vi "HFRR ADV v07.vi"() -> ()   [LabVIEW 2025] (continued)
                            n2274 = local write "EVENT LOG"(w3532) -> ()
                          }
                          frame Enabled {
                          }
                        }
                      }
                      frame #4 {
                        n2275 = Wait (ms)(milliseconds to wait=u32 50) -> ()  [unwired: 1 out]
                      }
                      frame #5 {
                        n2276 = local read "FILE"() -> (w3535:string)
                        n2277 = Concatenate Strings("File Name :" ("Content"), w3535) -> (w3536:string)
                        n2278 = local read "EVENT LOG"() -> (w3539:string)
                        n2279 = call "Event Log.vi"("Content"=w3536, "EVENT LOG"=w3539) -> ("EVENT LOG"=w3538:string)  [unwired: 8 in, 1 out]
                        n2280 = local write "EVENT LOG"(w3538) -> ()
                      }
                      frame #6 {
                        n2281 = Wait (ms)(milliseconds to wait=u32 50) -> ()  [unwired: 1 out]
                      }
                      frame #7 {
                        n2282 = local read "Batch Ref Num :"() -> (w3541:string)
                        n2283 = Concatenate Strings("Batch Ref No :" ("Content"), w3541) -> (w3542:string)
                        n2284 = local read "EVENT LOG"() -> (w3545:string)
                        n2285 = call "Event Log.vi"("Content"=w3542, "EVENT LOG"=w3545) -> ("EVENT LOG"=w3544:string)  [unwired: 8 in, 1 out]
                        n2286 = local write "EVENT LOG"(w3544) -> ()
                      }
                      frame #8 {
                        n2287 = Wait (ms)(milliseconds to wait=u32 50) -> ()  [unwired: 1 out]
                      }
                      frame #9 {
                        n2288 = local read "tested by"() -> (w3547:string)
                        n2289 = Concatenate Strings("Tested By :" ("Content"), w3547) -> (w3548:string)
                        n2290 = local read "EVENT LOG"() -> (w3551:string)
                        n2291 = call "Event Log.vi"("Content"=w3548, "EVENT LOG"=w3551) -> ("EVENT LOG"=w3550:string)  [unwired: 8 in, 1 out]
                        n2292 = local write "EVENT LOG"(w3550) -> ()
                      }
                      frame #10 {
                        n2293 = Wait (ms)(milliseconds to wait=u32 50) -> ()  [unwired: 1 out]
                      }
                      frame #11 {
                        n2294 = local read "TEST STANDARD"() -> (w3554:T4)
                        n2295 = case shown="\"ASTM D6079\", Default" w3554 {
                          tunnel: ["ASTM D6079" "ISO 12156" "CEC F-096-A-06" "Custom"] -> w3553
                          frame "ASTM D6079", Default {
                          }
                          frame "ISO 12156" {
                          }
                          frame "CEC F-096-A-06" {
                          }
                          frame "Custom" {
                          }
                        }
                        n2296 = Concatenate Strings("Test Standard :" ("Content"), w3553) -> (w3555:string)
                        n2297 = local read "EVENT LOG"() -> (w3558:string)
                        n2298 = call "Event Log.vi"("Content"=w3555, "EVENT LOG"=w3558) -> ("EVENT LOG"=w3557:string)  [unwired: 8 in, 1 out]
                        n2299 = local write "EVENT LOG"(w3557) -> ()
                      }
                      frame #12 {
                        n2300 = Wait (ms)(milliseconds to wait=u32 50) -> ()  [unwired: 1 out]
                      }
                      frame #13 {
                        n2301 = local read "Fuel Discription :"() -> (w3564:string)
                        n2302 = Concatenate Strings("Fuel Description :" ("Content"), w3564) -> (w3565:string)
                        n2303 = local read "EVENT LOG"() -> (w3568:string)
                        n2304 = call "Event Log.vi"("Content"=w3565, "EVENT LOG"=w3568) -> ("EVENT LOG"=w3567:string)  [unwired: 8 in, 1 out]
                        n2305 = local write "EVENT LOG"(w3567) -> ()
                      }
                      frame #14 {
                        n2306 = Wait (ms)(milliseconds to wait=u32 50) -> ()  [unwired: 1 out]
                      }
                      frame #15 {
                        n2307 = local read "Remarks :"() -> (w3570:string)
                        n2308 = Concatenate Strings("Remarks :" ("Content"), w3570) -> (w3571:string)
                        n2309 = local read "EVENT LOG"() -> (w3574:string)
                        n2310 = call "Event Log.vi"("Content"=w3571, "EVENT LOG"=w3574) -> ("EVENT LOG"=w3573:string)  [unwired: 8 in, 1 out]
                        n2311 = local write "EVENT LOG"(w3573) -> ()
                      }
                      frame #16 {
                        n2312 = Wait (ms)(milliseconds to wait=u32 50) -> ()  [unwired: 1 out]
                      }
                      frame #17 {
                        n2313 = local read "Operator ID"() -> (w3576:string)
                        n2314 = Concatenate Strings("Operator ID :" ("Content"), w3576) -> (w3578:string)
                        n2315 = local read "EVENT LOG"() -> (w3580:string)
                        n2316 = call "Event Log.vi"("Content"=w3578, "EVENT LOG"=w3580) -> ("EVENT LOG"=w3579:string)  [unwired: 8 in, 1 out]
                        n2317 = local write "EVENT LOG"(w3579) -> ()
                      }
                      frame #18 {
                        n2318 = Wait (ms)(milliseconds to wait=u32 50) -> ()  [unwired: 1 out]
                      }
                      frame #19 {
                        n2319 = disable-structure shown="Disabled" {
                          frame Disabled {
                            n2320 = local read "EVENT LOG"() -> (w3584:string)
                            n2321 = call "Event Log.vi"("Content"="Test Parameter", "EVENT LOG"=w3584) -> ("EVENT LOG"=w3583:string)  [unwired: 8 in, 1 out]
                            n2322 = local write "EVENT LOG"(w3583) -> ()
                          }
                          frame Enabled {
                          }
                        }
                      }
                      frame #20 {
                        n2323 = Wait (ms)(milliseconds to wait=u32 50) -> ()  [unwired: 1 out]
                      }
                      frame #21 {
                        n2324 = local read "Set Hz"() -> (w3588:dbl)
                        n2325 = Number To Fractional String(number=w3588, precision (6)=i16 2) -> (F-format string=w3587:string)  [unwired: 2 in]
                        n2326 = Concatenate Strings("Set Frequency [Hz] :" ("Content"), w3587) -> (w3590:string)
                        n2327 = local read "EVENT LOG"() -> (w3592:string)
                        n2328 = call "Event Log.vi"("Content"=w3590, "EVENT LOG"=w3592) -> ("EVENT LOG"=w3591:string)  [unwired: 8 in, 1 out]
                        n2329 = local write "EVENT LOG"(w3591) -> ()
                      }
                      frame #22 {
                        n2330 = Wait (ms)(milliseconds to wait=u32 50) -> ()  [unwired: 1 out]
                      }
                      frame #23 {
                        n2331 = local read "NORMAL LOAD"() -> (w3595:dbl)
                        n2332 = Number To Fractional String(number=w3595, precision (6)=i16 2) -> (F-format string=w3596:string)  [unwired: 2 in]
                        n2333 = Concatenate Strings("Applied Load [N] :" ("Content"), w3596) -> (w3598:string)
                        n2334 = local read "EVENT LOG"() -> (w3600:string)
                        n2335 = call "Event Log.vi"("Content"=w3598, "EVENT LOG"=w3600) -> ("EVENT LOG"=w3599:string)  [unwired: 8 in, 1 out]
                        n2336 = local write "EVENT LOG"(w3599) -> ()
                      }
                      frame #24 {
                        n2337 = Wait (ms)(milliseconds to wait=u32 50) -> ()  [unwired: 1 out]
                      }
                      frame #25 {
                        n2338 = local read "Set Strk"() -> (w3603:dbl)
                        n2339 = Number To Fractional String(number=w3603, precision (6)=i16 2) -> (F-format string=w3604:string)  [unwired: 2 in]
                        n2340 = Concatenate Strings("Set Stroke [mm] :" ("Content"), w3604) -> (w3606:string)
                        n2341 = local read "EVENT LOG"() -> (w3608:string)
                        n2342 = call "Event Log.vi"("Content"=w3606, "EVENT LOG"=w3608) -> ("EVENT LOG"=w3607:string)  [unwired: 8 in, 1 out]
                        n2343 = local write "EVENT LOG"(w3607) -> ()
                      }
                      frame #26 {
                        n2344 = Wait (ms)(milliseconds to wait=u32 50) -> ()  [unwired: 1 out]
                      }
                      frame #27 {
                        n2345 = local read "Set Temp"() -> (w3611:dbl)
                        n2346 = Number To Fractional String(number=w3611, precision (6)=i16 2) -> (F-format string=w3612:string)  [unwired: 2 in]
                        n2347 = Concatenate Strings("Set Temperature [deg C] :" ("Content"), w3612) -> (w3614:string)
                        n2348 = local read "EVENT LOG"() -> (w3616:string)
                        n2349 = call "Event Log.vi"("Content"=w3614, "EVENT LOG"=w3616) -> ("EVENT LOG"=w3615:string)  [unwired: 8 in, 1 out]
                        n2350 = local write "EVENT LOG"(w3615) -> ()
                      }
                      frame #28 {
                        n2351 = Wait (ms)(milliseconds to wait=u32 50) -> ()  [unwired: 1 out]
                      }
                      frame #29 {
                        n2352 = local read "Set Rh"() -> (w3619:dbl)
                        n2353 = Number To Fractional String(number=w3619, precision (6)=i16 2) -> (F-format string=w3620:string)  [unwired: 2 in]
                        n2354 = Concatenate Strings("Set Humidity [%RH] :" ("Content"), w3620) -> (w3622:string)
                        n2355 = local read "EVENT LOG"() -> (w3624:string)
                        n2356 = call "Event Log.vi"("Content"=w3622, "EVENT LOG"=w3624) -> ("EVENT LOG"=w3623:string)  [unwired: 8 in, 1 out]
                        n2357 = local write "EVENT LOG"(w3623) -> ()
                      }
                      frame #30 {
                        n2358 = Wait (ms)(milliseconds to wait=u32 50) -> ()  [unwired: 1 out]
                      }
                      frame #31 {
                        n2359 = local read "test time"() -> (w3627:dbl)
                        n2360 = Number To Fractional String(number=w3627, precision (6)=i16 1) -> (F-format string=w3628:string)  [unwired: 2 in]
                        n2361 = Concatenate Strings("Test Time [mins] :" ("Content"), w3628) -> (w3630:string)
                        n2362 = local read "EVENT LOG"() -> (w3632:string)
                        n2363 = call "Event Log.vi"("Content"=w3630, "EVENT LOG"=w3632) -> ("EVENT LOG"=w3631:string)  [unwired: 8 in, 1 out]
                        n2364 = local write "EVENT LOG"(w3631) -> ()
                      }
                    }
                  }
                }
              }
            }
          }
        }
        n2365 = case shown="True" w2932 {
          frame False {
            n2366 = local write "tfalg"(0.0 ("tfalg")) -> ()
          }
          frame True {
            n2367 = local read "tfalg"() -> (w3077:dbl)
            n2368 = Equal?(x=w3077, y=0.0) -> (x = y?=w3078:bool)
            n2369 = case shown="True" w3078 {
              frame False {
              }
              frame True {
                n2370 = local read "Total No. of Tests"() -> (w3081:dbl)
                n2371 = local write "tfalg"(1.0 ("tfalg")) -> ()
                n2372 = local write "acq 2"(FALSE ("acq 2")) -> ()
                n2373 = Wait (ms)(milliseconds to wait=u32 200) -> ()  [unwired: 1 out]
                n2374 = Increment(x=w3081) -> (x+1=w3080:dbl)
                n2375 = local write "Total No. of Tests"(w3080) -> ()
              }
            }
          }
        }
        n2376 = local write "Test \nStatus"(w2938) -> ()
        n2377 = local write "st enable"(w2938) -> ()
        n2378 = local write "PWR"(w2938) -> ()
        n2379 = local write "Save"(w2938) -> ()
        n2380 = local read "Main Tab"() -> (w2895:T3)
        n2381 = case shown="True" w2919 {
          tunnel: [FALSE ("RUN") TRUE ("RUN")] -> w2918
          tunnel: [_ 1] -> w2911
          frame False {
          }
          frame True {
          }
        }
        n2382 = In Range and Coerce(upper limit=w2926, x=w2899, lower limit=w2925) -> (In Range?=w2917:bool)  [unwired: 1 out]
        n2383 = In Range and Coerce(upper limit=w2923, x=w2898, lower limit=w2924) -> (In Range?=w2915:bool)  [unwired: 1 out]
        n2384 = case shown="True" w2931 {
          frame False {
            n2385 = local read "Rt 3"() -> (w3059:bool)
            n2386 = case shown="True" w3059 {
              frame False {
              }
              frame True {
                n2387 = local write "Rt 3"(FALSE ("Rt 3")) -> ()
                n2388 = local write "Json End Flg"(TRUE ("Upld AR 2")) -> ()
              }
            }
            "Rt" <- TRUE ("Rt")
            "Rt 2" <- FALSE ("Rt")
          }
          frame True {
            n2389 = local read "Rt"() -> (w3066:bool)
            n2390 = local write "Rt 2"(TRUE ("Rt 2")) -> ()
            n2391 = case shown="True" w3066 {
              frame False {
              }
              frame True {
                w3067 = TRUE ("Upld AR 2")
                n2392 = local write "Rt"(FALSE ("Rt")) -> ()
                n2393 = local write "Upld AR"(w3067) -> ()
                n2394 = local write "Json St Flg"(w3067) -> ()
              }
            }
            "Rt 3" <- TRUE ("Rt 3")
          }
        }
        n2395 = case shown="True" w2917 {
          tunnel: [FALSE ("RUN") TRUE ("RUN")] -> w2916
          tunnel: [_ 2] -> w2910
          frame False {
          }
          frame True {
          }
        }
        n2396 = case shown="True" w2915 {
          tunnel: [FALSE ("RUN") TRUE ("RUN")] -> w2914
          tunnel: [_ 3] -> w2909
          frame False {
          }
          frame True {
          }
        }
        n2397 = case shown="\"Acquire\"" w2895 {
          tunnel: w2897 -> [_ w3128]
          frame Default {
            w3127 = 0.0 ("output")
            n2398 = local write "PID-out"(w3127) -> ()
            n2399 = local write "Frequency ( Hz )"(w3127) -> ()
          }
          frame "Acquire" {
            n2400 = stacked-sequence {
              frame #0 {
                n2401 = local read "Auto Start Test"() -> (w3130:bool)
                n2402 = case shown="False" w3130 {
                  tunnel: "RUN" -> [w3151 w3154]
                  tunnel: [w3151 w3153] -> w3131
                  frame False {
                  }
                  frame True {
                    n2403 = local read "Auto Start Temp"() -> (w3152:bool)
                    n2404 = Or(x=w3154, y=w3152) -> (x .or. y?=w3153:bool)
                  }
                }
                n2405 = local read "clk"() -> (w3150:dbl)
                n2406 = local read "Save"() -> (w3146:bool)
                n2407 = Equal?(x=w3150, y=0.0) -> (x = y?=w3147:bool)
                n2408 = And(x=w3147, y=w3146) -> (x .and. y?=w3148:bool)
                n2409 = Not(x="Engage") -> (.not. x?=w3137:bool)
                n2410 = case shown="False" w3131 {
                  tunnel: [w3163 w3179] -> w3133
                  frame False {
                    w3163 = 0.0
                    n2411 = local write "Reinit PID"(TRUE) -> ()
                    n2412 = local write "Start Time"(TRUE ("Start Time")) -> ()
                    n2413 = property on="Stroke" class="DigNum (strict)"("Visible"=TRUE) -> ()  [unwired: 2 in, 2 out]
                    n2414 = property on="Stroke 2" class="DigNum (strict)"("Visible"=FALSE) -> ()  [unwired: 2 in, 2 out]
                    n2415 = property on="Heater Button" class="Bool (strict)"("DisabledEnum"=T15."Enabled" ("Disabled")) -> ()  [unwired: 2 in, 2 out]
                    n2416 = property on="Humidity" class="Bool (strict)"("DisabledEnum"=T15."Enabled" ("Disabled")) -> ()  [unwired: 2 in, 2 out]
                    n2417 = case shown="False" "TestCompFlg" {
                      frame False {
                        n2418 = local read "StartFlg"() -> (w3167:bool)
                        n2419 = case shown="True" w3167 {
                          frame False {
                          }
                          frame True {
                            n2420 = flat-sequence {
                              frame #0 {
                                n2421 = local read "EVENT LOG"() -> (w3169:string)
                                n2422 = call "Event Log.vi"("Content"="Test was interrupted", "EVENT LOG"=w3169) -> ("EVENT LOG"=w3170:string)  [unwired: 8 in, 1 out]
                                n2423 = local write "EVENT LOG"(w3170) -> ()
                              }
                              frame #1 {
                                w3171 = FALSE ("StartFlg")
                                n2424 = local write "Heater Button"(w3171) -> ()
                                n2425 = local write "StartFlg"(w3171) -> ()
                                n2426 = local write "Humidity"(w3171) -> ()
                              }
                            }
                          }
                        }
                      }
                      frame True {
                      }
                    }
                    n2427 = local write "String 14"("Test will autostart once parameters reach the set value." ("String 14")) -> ()
                    n2428 = local write "Old Pid Val"(w3163) -> ()
                  }
                  frame True {
                    n2429 = property on="Stroke 2" class="DigNum (strict)"("Visible"=TRUE) -> ()  [unwired: 2 in, 2 out]
                    n2430 = property on="Stroke" class="DigNum (strict)"("Visible"=FALSE) -> ()  [unwired: 2 in, 2 out]
                    n2431 = property on="STOP 2" class="Bool (strict)"("Disabled"=u8 2) -> ()  [unwired: 2 in, 2 out]
                    n2432 = local write "String 14"(" Running....." ("String 14")) -> ()
                    n2433 = property on="Heater Button" class="Bool (strict)"("DisabledEnum"=T15."Disabled and Grayed Out" ("Disabled")) -> ()  [unwired: 2 in, 2 out]
                    n2434 = property on="Humidity" class="Bool (strict)"("DisabledEnum"=T15."Disabled and Grayed Out" ("Disabled")) -> ()  [unwired: 2 in, 2 out]
                    n2435 = local read "PID Ref"() -> (w3190:bool)
                    n2436 = case shown="True" w3190 {
                      tunnel: [w3196 w3212] -> w3189
                      frame False {
                        n2437 = local read "Old Pid Val"() -> (w3196:dbl)
                      }
                      frame True {
                        n2438 = local read "Set Hz"() -> (w3205:dbl)
                        n2439 = local read "Frequency"() -> (w3216:dbl)
                        n2440 = Add(x=w3205, y=10.0) -> (x+y=w3214:dbl)
                        n2441 = Add(x=w3205, y=-10.0 ("Offset")) -> (x+y=w3223:dbl)
                        n2442 = Add(x=w3205, y=-10.0) -> (x+y=w3215:dbl)
                        n2443 = In Range and Coerce(upper limit=w3214, x=w3216, lower limit=w3215) -> (coerced(x)=w3204:dbl)  [unwired: 1 out]
                        n2444 = Or(x="Reinit PID", y="Reinit PID") -> (x .or. y?=w3213:bool)
                        n2445 = Multiply(x=w3223, y=0.1 ("Gain")) -> (x*y=w3202:dbl)
                        n2446 = local read "Elapsed time"() -> (w3209:dbl)
                        n2447 = local read "SPEED OUT:"() -> (w3224:dbl)
                        n2448 = Add(x=w3202, y=1.5) -> (x+y=w3200:dbl)
                        n2449 = call-poly <vilib>:"PID.vi"("reinitialize? (F)"=w3213, "output range"=cluster{"output high":dbl, "output low":dbl} {"output high"=1.0, "output low"=-1.0}, "PID gains"=T11 {"proportional gain (Kc)"=0.0005, "integral time (Ti, min)"=0.001, "derivative time (Td, min)"=0.0} ("Motor PID"), "process variable"=w3204, "setpoint"=w3205) -> ("output"=w3203:dbl)  [unwired: 5 in, 1 out]
                        n2450 = Multiply(x=w3200, y=w3224) -> (x*y=w3199:dbl)
                        n2451 = Greater?(x=w3209, y=0.05) -> (0:w3208:bool)
                        n2452 = case shown="True" w3208 {
                          tunnel: w3203 -> [_ w3226]
                          tunnel: [0.0 ("output") w3226] -> w3206
                          frame False {
                          }
                          frame True {
                            n2453 = local write "Reinit PID"(FALSE ("Reinit PID")) -> ()
                          }
                        }
                        n2454 = Multiply(x=w3199, y=0.8) -> (x*y=w3198:dbl)
                        n2455 = Add(x=w3198, y=w3206) -> (x+y=w3211:dbl)
                        n2456 = flat-sequence {
                          tunnel: [w3229] -> w3212
                          tunnel: w3211 -> [w3229]
                          frame #0 {
                            n2457 = local write "PID Ref"(FALSE ("PID Ref")) -> ()
                          }
                        }
                      }
                    }
                    "Old Pid Val" <- w3189
                    n2458 = case shown="False" "Start Time" {
                      selector: "Start Time" -> [_ w3192]
                      frame False {
                      }
                      frame True {
                        n2459 = Not(x=w3192) -> (.not. x?=w3191:bool)
                        n2460 = local write "Start Time"(w3191) -> ()
                        n2461 = local read "EVENT LOG"() -> (w3193:string)
                        n2462 = call "Event Log.vi"("Content"="Test in progress", "EVENT LOG"=w3193) -> ("EVENT LOG"=w3195:string)  [unwired: 8 in, 1 out]
                        n2463 = local write "EVENT LOG"(w3195) -> ()
                      }
                    }
                    n2464 = local read "Set Hz"() -> (w3186:dbl)
                    n2465 = call <vilib>:"Uniform White Noise Waveform.vi"() -> ("signal out"=w3185:waveform(dbl))  [unwired: 10 in, 1 out]
                    n2466 = local read "Freq"() -> (w3178:dbl)
                    n2467 = Add(x=w3186, y=w3185) -> (x+y=w3184:waveform(dbl))
                    n2468 = Multiply(x=w3184, y=ext 0.1) -> (x*y=w3180:waveform(ext))
                    n2469 = Multiply(x=w3178, y=0.9) -> (x*y=w3181:dbl)
                    n2470 = Add(x=w3180, y=w3181) -> (x+y=w3179:waveform(ext))
                    "StartFlg" <- TRUE ("StartFlg")
                  }
                }
                n2471 = case shown="True" w3148 {
                  frame False {
                  }
                  frame True {
                    n2472 = local write "clk"(10.0 ("clk")) -> ()
                    n2473 = Get Date/Time In Seconds() -> (seconds since 1Jan1904=w3232:timestamp)
                    n2474 = To Double Precision Float(number=w3232) -> (double precision float=w3230:dbl)
                    n2475 = local write "acq timer"(w3230) -> ()
                    n2476 = local write "act save time"(w3230) -> ()
                  }
                }
                n2477 = call "Elapsed Time"("Time Target (s)"="Countdown", "Reset"=w3137) -> ("Elapsed Time (s)"=w3142:dbl, "Time has Elapsed"=w3140:bool)  [unwired: 10 in, 6 out]
                "Countdown 2" <- w3142
                n2478 = Subtract(x=w3142, y=2.0) -> (x-y=w3145:dbl)
                n2479 = Less?(x=w3145, y="Countdown") -> (x < y?=w3143:bool)
                n2480 = And(x=w3143, y=w3140) -> (x .and. y?=w3139:bool)
                n2481 = case shown="True" w3139 {
                  frame False {
                  }
                  frame True {
                    (unwired) dbl[] [] ("History Data")
                    n2482 = local write "Engage"(FALSE ("Engage")) -> ()
                    n2483 = local write "RUN"(TRUE ("RUN")) -> ()
                    n2484 = local read "Humidity ( %RH )"() -> (→"Rh Before":dbl)
                  }
                }
                n2485 = local read "Test \nStatus"() -> (w3135:bool)
                n2486 = Select(t=w3133, s=w3135, f=0.0) -> (s? t:f=w3134:dbl)
                n2487 = local write "Frequency ( Hz )"(w3134) -> ()
                n2488 = local write "Freq"(w3134) -> ()
              }
              frame #1 {
                w3255 = 1000000.0 ("x")
                # "Elapsed time\ncof\nstroke\nAir temp\nTemp\nHumidity"
                # "acq timer\n\nact save time"
                # "convert to microseconds"
                n2489 = local read "COUNT"() -> (w3238:i32)
                n2490 = local read "Rate"() -> (w3251:dbl)
                n2491 = Divide(x=w3255, y=w3251) -> (x/y=w3256:dbl)
                n2492 = Greater Or Equal?(x=w3238, y=250) -> (x >= y?=w3237:bool)
                n2493 = Get Date/Time In Seconds() -> (seconds since 1Jan1904=w3258:timestamp)
                n2494 = case shown="True" w3237 {
                  frame False {
                    n2495 = local read "COUNT"() -> (w3259:i32)
                    n2496 = Increment(x=w3259) -> (x+1=w3260:i32)
                    n2497 = local write "COUNT"(w3260) -> ()
                  }
                  frame True {
                    n2498 = local write "COUNT"(0 ("COUNT")) -> ()
                  }
                }
                n2499 = local read "Samplingtime 2"() -> (w3236:dbl)
                n2500 = local read "act save time"() -> (w3253:dbl)
                n2501 = Divide(x=w3256, y=w3255) -> (x/y=w3254:dbl)
                n2502 = To Double Precision Float(number=w3258) -> (double precision float=w3247:dbl)
                n2503 = Add(x=w3253, y=w3236) -> (x+y=w3252:dbl)
                n2504 = local read "acq timer"() -> (w3257:dbl)
                n2505 = local read "COUNT"() -> (w3240:i32)
                n2506 = Greater Or Equal?(x=w3247, y=w3252) -> (x >= y?=w3235:bool)
                n2507 = Multiply(x=w3254, y=w3240) -> (x*y=w3246:dbl)
                n2508 = Subtract(x=w3247, y=w3257) -> (x-y=w3249:dbl)
                n2509 = local read "Save"() -> (w3250:bool)
                n2510 = Add(x=w3249, y=w3246) -> (x+y=w3233:dbl)
                "Elapsed time 3" <- w3233
                n2511 = And(x=w3235, y=w3250) -> (x .and. y?=w3248:bool)
                n2512 = Divide(x=w3233, y=60.0) -> (x/y=w3244:dbl)
                n2513 = local read "Test \nStatus"() -> (w3234:bool)
                n2514 = local read "clk"() -> (w3241:dbl)
                n2515 = Equal?(x=w3241, y=10.0) -> (x = y?=w3243:bool)
                n2516 = case shown="True" w3248 {
                  tunnel: w3247 -> [_ w3354]
                  tunnel: [FALSE ("Boolean 2") TRUE ("Boolean 2")] -> _
                  frame False {
                  }
                  frame True {
                    w3301 = ";" ("Substring")
                    # "Pid out/\nFreq response value"
                    n2517 = local write "act save time"(w3354) -> ()
                    n2518 = local read "FILE"() -> (w3295:string)
                    n2519 = call "file check.vi"("file name in"=w3295) -> ("error out"=w3298:errorcluster, "file name out"=w3293:string)  [unwired: 9 in]
                    n2520 = call "FILE PATH CREATION.vi"("error in"=w3298, "FILE NAME :"=w3293) -> ("FILE OUT"=w3296:path)  [unwired: 8 in, 1 out]
                    n2521 = Concatenate Strings(w3293, ".dgf" ("Substring")) -> (w3297:string)
                    n2522 = local read "Set Strk"() -> (w3325:dbl)
                    n2523 = local read "Stroke"() -> (w3316:dbl)
                    n2524 = local read "FF 2"() -> (w3312:dbl)
                    "Frictional Force ( N )" <- w3312
                    "Frictional Force ( N )" <- w3312
                    n2525 = Build Path(base path=w3296, name or relative path=w3297) -> (appended path=w3292:path)
                    n2526 = local write "FF 3"(w3312) -> ()
                    n2527 = Subtract(x=w3316, y=w3325) -> (x-y=w3322:dbl)
                    n2528 = local read "COF 2"() -> (w3307:dbl)
                    "cof" <- w3307
                    "Coefficient of Friction" <- w3307
                    "COF 4" <- w3307
                    "Coefficient of Friction" <- w3307
                    n2529 = local write "COF 3"(w3307) -> ()
                    n2530 = Multiply(x=w3322, y=0.05) -> (x*y=w3324:dbl)
                    n2531 = local read "TEMP"() -> (w3311:dbl)
                    "Temp" <- w3311
                    "Temperature ( Deg C )" <- w3311
                    n2532 = Add(x=w3324, y=w3325) -> (x+y=w3305:dbl)
                    "Stroke Ln" <- w3305
                    "Disp" <- w3305
                    n2533 = local read "ecr"() -> (w3308:dbl)
                    "ecr 2" <- w3308
                    "Electrical Contact Resistance ( % )" <- w3308
                    "ecr 4" <- w3308
                    n2534 = local read "Humidity ( %RH )"() -> (w3310:dbl)
                    "Humidity ( %RH )" <- w3310
                    "Humidity ( %RH )" <- w3310
                    n2535 = local read "Frequency ( Hz )"() -> (w3318:dbl)
                    n2536 = local read "Elapsed time"() -> (w3347:dbl)
                    n2537 = local read "AIR TEMP"() -> (w3315:dbl)
                    n2538 = local write "ecr 3"(w3308) -> ()
                    n2539 = local read "PID-out"() -> (w3321:dbl)
                    n2540 = local write "Temperature ( Deg C )"(w3311) -> ()
                    n2541 = local write "Electrical Contact Resistance ( % )"(w3308) -> ()
                    n2542 = Number To Fractional String(number=w3305, width (-)=i16 9 ("precision (6)"), precision (6)=i16 6) -> (F-format string=w3340:string)  [unwired: 1 in]
                    n2543 = Number To Fractional String(number=w3315, width (-)=i16 9 ("precision (6)"), precision (6)=i16 3) -> (F-format string=w3339:string)  [unwired: 1 in]
                    n2544 = Number To Fractional String(number=w3311, width (-)=i16 9 ("precision (6)"), precision (6)=i16 3) -> (F-format string=w3336:string)  [unwired: 1 in]
                    n2545 = Number To Fractional String(number=w3310, width (-)=i16 9 ("precision (6)"), precision (6)=i16 3) -> (F-format string=w3333:string)  [unwired: 1 in]
                    n2546 = Number To Fractional String(number=w3308, width (-)=i16 9 ("precision (6)"), precision (6)=i16 3) -> (F-format string=w3330:string)  [unwired: 1 in]
                    n2547 = Number To Fractional String(number=w3321, width (-)=i16 9 ("precision (6)"), precision (6)=i16 3) -> (F-format string=w3326:string)  [unwired: 1 in]
                    n2548 = Number To Fractional String(number=w3318, width (-)=i16 9 ("precision (6)"), precision (6)=i16 3) -> (F-format string=w3317:string)  [unwired: 1 in]
                    n2549 = Number To Fractional String(number=w3307, width (-)=i16 9 ("precision (6)"), precision (6)=i16 6) -> (F-format string=w3348:string)  [unwired: 1 in]
                    n2550 = Number To Fractional String(number=w3347, width (-)=i16 14 ("precision (6)"), precision (6)=i16 3) -> (F-format string=w3349:string)  [unwired: 1 in]
                    n2551 = Bundle("y"=1.02, w3305, "y"=0.98) -> (w3309:cluster{"y":dbl, dbl, "y":dbl})  [unwired: 1 in]
                    n2552 = Number To Fractional String(number="Ambient Humidity :", width (-)=i16 9 ("precision (6)"), precision (6)=i16 6) -> (F-format string=w3299:string)  [unwired: 1 in]
                    n2553 = local read "RUN"() -> (w3306:bool)
                    n2554 = case shown="True" w3306 {
                      tunnel: w3309 -> [_ w3359]
                      tunnel: w3305 -> [_ w3358]
                      tunnel: w3305 -> [_ w3357]
                      tunnel: w3305 -> [_ w3356]
                      frame False {
                      }
                      frame True {
                        "Stroke ( mm )" <- w3359
                        "Stroke ( mm )" <- w3359
                        "Stroke 4" <- w3358
                        "Stroke 3" <- w3357
                        "Stroke 2" <- w3356
                      }
                    }
                    n2555 = Concatenate Strings(w3349, w3301, w3348, w3301, w3340, w3301, w3339, w3301, w3336, w3301, w3333, w3301, w3330, w3301, w3326, w3301, w3317, w3301, w3299, "\r") -> (w3346:string)
                    n2556 = call <vilib>:"Write Characters To File.vi"("append to file? (new file:F)"=TRUE, "character string"=w3346, "file path (dialog if empty)"=w3292) -> ()  [unwired: 2 in, 1 out]
                    "refresh flag" <- TRUE ("refresh flag")
                  }
                }
                n2557 = case shown="True" w3234 {
                  tunnel: w3244 -> [_ w3267]
                  tunnel: w3249 -> [_ w3278]
                  tunnel: [0.0 w3274] -> _
                  tunnel: w3243 -> [_ w3273]
                  tunnel: [0.0 w3272] -> _
                  tunnel: w3233 -> [_ w3272]
                  tunnel: w3247 -> [w3263 _]
                  frame False {
                    n2558 = local write "acq timer"(w3263) -> ()
                    n2559 = local write "Test Duration Status"(0.0 ("Test Duration Status")) -> ()
                  }
                  frame True {
                    n2560 = local read "Set Hz"() -> (w3275:dbl)
                    n2561 = local write "Elapsed time"(w3267) -> ()
                    n2562 = local read "test time"() -> (w3266:dbl)
                    n2563 = Multiply(x=w3278, y=w3275) -> (x*y=w3277:dbl)
                    n2564 = case shown="False" w3273 {
                      tunnel: w3277 -> [w3279 _]
                      tunnel: [w3279 1.0] -> w3274
                      frame False {
                        n2565 = local write "Cycles elapsed"(w3279) -> ()
                      }
                      frame True {
                      }
                    }
                    n2566 = Greater?(x=w3267, y=w3266) -> (0:w3276:bool)
                    n2567 = Subtract(x=w3266, y=w3267) -> (x-y=w3271:dbl)
                    "time" <- w3271
                    n2568 = local write "Time Remaining"(w3271) -> ()
                    n2569 = case shown="True" w3276 {
                      frame False {
                      }
                      frame True {
                        n2570 = local write "Humidity"(FALSE ("Humidity")) -> ()
                        n2571 = local write "RUN"(FALSE ("OK Button 2")) -> ()
                        n2572 = local write "Heater Button"(FALSE ("Heater Button")) -> ()
                        n2573 = local write "Auto Start Test"(FALSE ("Auto Start Test")) -> ()
                        n2574 = local write "TestCompFlg"(TRUE ("StpFlg")) -> ()
                        n2575 = local read "Humidity ( %RH )"() -> (→"Rh After":dbl)
                        n2576 = property on="STOP 2" class="Bool (strict)"("Disabled"=u8 0) -> ()  [unwired: 2 in, 2 out]
                        n2577 = local read "EVENT LOG"() -> (w3285:string)
                        n2578 = call "Event Log.vi"("Content"="Test Completed", "EVENT LOG"=w3285) -> ("EVENT LOG"=w3284:string)  [unwired: 8 in, 1 out]
                        n2579 = local write "EVENT LOG"(w3284) -> ()
                      }
                    }
                    n2580 = Divide(x=w3267, y=w3266) -> (x/y=w3270:dbl)
                    n2581 = Multiply(x=w3270, y=100.0) -> (x*y=w3268:dbl)
                    n2582 = local write "Test Duration Status"(w3268) -> ()
                  }
                }
              }
              frame #2 {
                n2583 = case shown="True" "Heater Button" {
                  tunnel: [0.0 ("output") w3383] -> w3360
                  frame False {
                    w3363 = TRUE ("tmpchk")
                    n2584 = local read "TEMP"() -> (w3364:dbl)
                    n2585 = local write "Temp ini"(w3364) -> ()
                    n2586 = local write "Reset 4"(w3363) -> ()
                    n2587 = local write "tmpchk"(w3363) -> ()
                    n2588 = local write "reinit"(TRUE ("reinit")) -> ()
                    n2589 = local write "manual temp log"(TRUE ("manual temp log")) -> ()
                  }
                  frame True {
                    # "Logic to turn off\nthe heater when \ntemp is not rising.\nTime - 60 sec\nDelta t- 5°c"
                    n2590 = local read "Temp ini"() -> (w3371:dbl)
                    n2591 = local read "Auto Start Test"() -> (w3367:bool)
                    n2592 = Less?(x=w3371, y=53.0) -> (x < y?=w3369:bool)
                    n2593 = case shown="False" w3367 {
                      frame False {
                        n2594 = local read "Set Temp"() -> (w3394:dbl)
                        n2595 = local read "TEMP"() -> (w3393:dbl)
                        n2596 = Subtract(x=w3394, y=w3393) -> (x-y=w3392:dbl)
                        n2597 = Absolute Value(x=w3392) -> (abs(x)=w3391:dbl)
                        n2598 = Less?(x=w3391, y=0.5) -> (x < y?=w3389:bool)
                        n2599 = case shown="True" w3389 {
                          tunnel: "manual temp log" -> [_ w3395]
                          frame False {
                          }
                          frame True {
                            n2600 = case shown="True" w3395 {
                              selector: w3395 -> [_ w3396]
                              frame False {
                              }
                              frame True {
                                # "#Event log"
                                n2601 = Not(x=w3396) -> (.not. x?=w3397:bool)
                                n2602 = local write "manual temp log"(w3397) -> ()
                                n2603 = local read "EVENT LOG"() -> (w3400:string)
                                n2604 = call "Event Log.vi"("Content"="Target Temperature reached", "EVENT LOG"=w3400) -> ("EVENT LOG"=w3399:string)  [unwired: 8 in, 1 out]
                                n2605 = local write "EVENT LOG"(w3399) -> ()
                              }
                            }
                          }
                        }
                      }
                      frame True {
                        n2606 = local write "manual temp log"(TRUE ("manual temp log")) -> ()
                      }
                    }
                    n2607 = And(x="tmpchk", y=w3369) -> (x .and. y?=w3372:bool)
                    n2608 = case shown="True" w3372 {
                      frame False {
                      }
                      frame True {
                        n2609 = call "Elapsed Time8"("Time Target (s)"=300.0, "Reset"="Reset 4") -> ("Time has Elapsed"=w3402:bool)  [unwired: 10 in, 7 out]
                        n2610 = flat-sequence {
                          tunnel: w3402 -> [_]
                          frame #0 {
                            n2611 = local write "Reset 4"(FALSE ("Reset 4")) -> ()
                          }
                        }
                        n2612 = case shown="True" w3402 {
                          frame False {
                          }
                          frame True {
                            n2613 = local read "Temp ini"() -> (w3409:dbl)
                            n2614 = Add(x=w3409, y=5.0) -> (x+y=w3407:dbl)
                            n2615 = local read "TEMP"() -> (w3410:dbl)
                            n2616 = Greater?(x=w3410, y=w3407) -> (0:w3408:bool)
                            n2617 = case shown="False" w3408 {
                              frame False {
                                n2618 = local write "Heater Button"(FALSE ("Heater Button")) -> ()
                              }
                              frame True {
                                n2619 = local write "tmpchk"(FALSE ("tmpchk")) -> ()
                              }
                            }
                          }
                        }
                      }
                    }
                    n2620 = local read "Set Temp"() -> (w3380:dbl)
                    n2621 = local read "TEMP"() -> (w3374:dbl)
                    n2622 = call-poly <vilib>:"PID.vi"("reinitialize? (F)"="reinit", "output range"="output range", "dt (s)"=-1.0, "PID gains"="Temp PID gains", "process variable"=w3374, "setpoint"=w3380) -> ("output"=w3377:dbl)  [unwired: 4 in, 1 out]
                    n2623 = Subtract(x=w3380, y=w3374) -> (x-y=w3382:dbl)
                    n2624 = Add(x=w3380, y=0.5) -> (x+y=w3378:dbl)
                    n2625 = Greater Or Equal?(x=w3374, y=w3378) -> ()  [unwired: 1 out]
                    n2626 = Select(t=0.0, s=FALSE, f=w3377) -> (s? t:f=w3376:dbl)
                    "PID output" <- w3376
                    n2627 = flat-sequence {
                      tunnel: w3376 -> [w3413]
                      tunnel: [w3413] -> w3383
                      frame #0 {
                        n2628 = local write "reinit"(FALSE ("reinit")) -> ()
                      }
                    }
                    n2629 = Bundle(w3382, "output"=w3376, "TEMP"=w3374) -> (→"gTEMP 3":cluster{dbl, "output":dbl, "TEMP":dbl})  [unwired: 1 in]
                  }
                }
                "PID-out" <- w3360
              }
              frame #3 {
                n2630 = local read "TEMP"() -> (w3415:dbl)
                n2631 = Greater Or Equal?(x=w3415, y="Set Temp 2") -> (x >= y?=w3420:bool)
                n2632 = case shown="True" w3420 {
                  tunnel: [FALSE TRUE] -> w3418
                  frame False {
                  }
                  frame True {
                  }
                }
                "Status 13" <- w3418
                n2633 = And(x=w3418, y="trip1 8") -> (x .and. y?=w3417:bool)
                n2634 = case shown="True" w3417 {
                  frame False {
                  }
                  frame True {
                    w3421 = FALSE ("OK Button 2")
                    n2635 = local write "RUN"(w3421) -> ()
                    n2636 = local write "Heater Button"(w3421) -> ()
                  }
                }
              }
            }
            n2637 = case shown="False" w3128 {
              frame False {
                n2638 = disable-structure shown="Enabled" {
                  frame Enabled {
                    n2639 = stacked-sequence {
                      frame #0 {
                        n2640 = local write "RUN"(FALSE ("OK Button 2")) -> ()
                      }
                      frame #1 {
                      }
                    }
                  }
                  frame Disabled {
                  }
                }
              }
              frame True {
              }
            }
          }
        }
        n2641 = local read "airtempflg"() -> (w2920:bool)
        n2642 = Or(x=w2920, y=w2918) -> (x .or. y?=w2921:bool)
        n2643 = Insert Into Array(array=string[] ["Air Temperature has reached set value,", "Humidity has reached set value,", "Sample Temperaturehas reached set value,", ""], index=0, new element="") -> (w2906:string[])
        n2644 = Build Array(w2911, w2910, w2909) -> (w2907:i32[])
        n2645 = disable-structure shown="Disabled" {
          disable-tunnel: w2921 -> [w2998 _]
          disable-tunnel: w2916 -> [w2997 _]
          disable-tunnel: w2914 -> [w2996 _]
          frame Disabled {
            n2646 = Compound Arithmetic op=AND(w2998, w2997, w2996) -> ()  [unwired: 1 out]
            n2647 = case shown="True" {
              selector: _ -> [_ _]
              frame False {
              }
              frame True {
                w2999 = FALSE ("autostrtflg")
                n2648 = local write "RUN"(TRUE ("RUN")) -> ()
                n2649 = local write "autostrtflg"(w2999) -> ()
                n2650 = local write "autostart"(w2999) -> ()
                n2651 = local write "String 14"(" Running....." ("String 14")) -> ()
              }
            }
          }
          frame Enabled {
          }
        }
        n2652 = for {
          tunnel: w2907 -> [w3049] mode=indexing
          tunnel: w2906 -> [w3048]
          shift-right: [w3045] -> w2905
          shift-left: "" -> [w3047]
          n2653 = Index Array(array=w3048, index=w3049) -> (element=w3046:string)
          n2654 = Concatenate Strings(w3046, w3047) -> (w3045:string)
        }
        n2655 = local write "autostart 2"(w2905) -> ()
        n2656 = local read "Reset Graph"() -> (w2894:bool)
        n2657 = case shown="True" w2894 {
          selector: w2894 -> [_ w2948]
          frame False {
          }
          frame True {
            w2962 = 0.0 ("X Scale.Range:Maximum")
            n2658 = Not(x=w2948) -> (.not. x?=w2947:bool)
            n2659 = local write "Reset Graph"(w2947) -> ()
            n2660 = property on="Electrical Contact Resistance ( % )" class="WFChart (strict)"("XScale.Maximum"=600.0 ("X Scale.Range:Maximum"), "XScale.Minimum"=0.0 ("X Scale.Range:Minimum"), "YScale.Maximum"=100.0 ("Y Scale.Range:Maximum"), "YScale.Minimum"=0.0 ("Y Scale.Range:Minimum")) -> ()  [unwired: 2 in, 2 out]
            n2661 = property on="Frictional Force ( N )" class="WFChart (strict)"("XScale.Maximum"=600.0 ("X Scale.Range:Maximum"), "XScale.Minimum"=0.0 ("X Scale.Range:Minimum"), "YScale.Maximum"=100.0 ("Y Scale.Range:Maximum"), "YScale.Minimum"=0.0 ("Y Scale.Range:Minimum")) -> ()  [unwired: 2 in, 2 out]
            n2662 = property on="Temperature ( Deg C )" class="WFChart (strict)"("XScale.Maximum"=600.0 ("X Scale.Range:Maximum"), "XScale.Minimum"=0.0 ("X Scale.Range:Minimum"), "YScale.Maximum"=100.0 ("Y Scale.Range:Maximum"), "YScale.Minimum"=0.0 ("Y Scale.Range:Minimum")) -> ()  [unwired: 2 in, 2 out]
            n2663 = property on="Humidity ( %RH )" class="WFChart (strict)"("XScale.Maximum"=600.0 ("X Scale.Range:Maximum"), "XScale.Minimum"=0.0 ("X Scale.Range:Minimum"), "YScale.Maximum"=100.0 ("Y Scale.Range:Maximum"), "YScale.Minimum"=0.0 ("Y Scale.Range:Minimum")) -> ()  [unwired: 2 in, 2 out]
            n2664 = property on="Stroke ( mm )" class="WFChart (strict)"("XScale.Maximum"=600.0 ("X Scale.Range:Maximum"), "XScale.Minimum"=0.0 ("X Scale.Range:Minimum"), "YScale.Maximum"=100.0 ("Y Scale.Range:Maximum"), "YScale.Minimum"=0.0 ("Y Scale.Range:Minimum")) -> ()  [unwired: 2 in, 2 out]
            n2665 = property on="Coefficient of Friction" class="WFChart (strict)"("XScale.Maximum"=600.0 ("X Scale.Range:Maximum"), "XScale.Minimum"=0.0 ("X Scale.Range:Minimum"), "YScale.Maximum"=100.0 ("Y Scale.Range:Maximum"), "YScale.Minimum"=0.0 ("Y Scale.Range:Minimum")) -> ()  [unwired: 2 in, 2 out]
            n2666 = property on="Electrical Contact Resistance ( % )" class="WFChart (strict)"("XScale.Minimum"=0.0 ("X Scale.Range:Minimum"), "XScale.Maximum"=600.0 ("X Scale.Range:Maximum"), "YScale.Minimum"=0.0 ("Y Scale.Range:Minimum"), "YScale.Maximum"=100.0 ("Y Scale.Range:Maximum")) -> ()  [unwired: 2 in, 2 out]
            n2667 = property on="Temperature ( Deg C )" class="WFChart (strict)"("XScale.Minimum"=0.0 ("X Scale.Range:Minimum"), "XScale.Maximum"=600.0 ("X Scale.Range:Maximum"), "YScale.Minimum"=0.0 ("Y Scale.Range:Minimum"), "YScale.Maximum"=100.0 ("Y Scale.Range:Maximum")) -> ()  [unwired: 2 in, 2 out]
            n2668 = property on="Coefficient of Friction" class="WFChart (strict)"("XScale.Minimum"=0.0 ("X Scale.Range:Minimum"), "XScale.Maximum"=600.0 ("X Scale.Range:Maximum"), "YScale.Maximum"=1.0 ("X Scale.Range:Minimum"), "YScale.Minimum"=0.0 ("X Scale.Range:Minimum")) -> ()  [unwired: 2 in, 2 out]
            n2669 = property on="Frictional Force ( N )" class="WFChart (strict)"("XScale.Maximum"=600.0 ("X Scale.Range:Maximum"), "XScale.Minimum"=w2962, "YScale.Maximum"=10.0 ("Y Scale.Range:Maximum"), "YScale.Minimum"=w2962) -> ()  [unwired: 2 in, 2 out]
            n2670 = property on="Stroke ( mm )" class="WFChart (strict)"("XScale.Maximum"=600.0 ("X Scale.Range:Maximum"), "XScale.Minimum"=0.0 ("X Scale.Range:Minimum"), "YScale.Maximum"=100.0 ("Y Scale.Range:Maximum"), "YScale.Minimum"=0.0 ("Y Scale.Range:Minimum")) -> ()  [unwired: 2 in, 2 out]
            n2671 = property on="Humidity ( %RH )" class="WFChart (strict)"("XScale.Maximum"=600.0 ("X Scale.Range:Maximum"), "XScale.Minimum"=0.0 ("X Scale.Range:Minimum"), "YScale.Maximum"=100.0 ("Y Scale.Range:Maximum"), "YScale.Minimum"=0.0 ("Y Scale.Range:Minimum")) -> ()  [unwired: 2 in, 2 out]
          }
        }
      }
      frame "Compare Files" {
        # "Elapsed time\ncof\nstroke\nAir temp\nTemp\nHumidity"
        n2672 = case shown="True" "RSTV1 2" {
          frame False {
          }
          frame True {
            n2673 = property on="Humidity ( %RH )" class="XYGraph (strict)"("Y Scale.Display Format:Precision"=u8 0 ("Y Scale.Format & Precision:Precision")) -> ()  [unwired: 2 in, 2 out]
            n2674 = property on="Humidity ( %RH )" class="XYGraph (strict)"("X Scale.Range:Minimum"=0.0, "X Scale.Range:Maximum"=75.0, "Y Scale.Range:Minimum"=48.0, "Y Scale.Range:Maximum"=58.0) -> ()  [unwired: 2 in, 2 out]
          }
        }
        n2675 = case shown="True" "RST CP 2" {
          frame False {
          }
          frame True {
            n2676 = property on="XY Graph 13" class="XYGraph (strict)"("Y Scale.Display Format:Precision"=u8 0 ("Y Scale.Format & Precision:Precision")) -> ()  [unwired: 2 in, 2 out]
            n2677 = property on="XY Graph 13" class="XYGraph (strict)"("X Scale.Range:Minimum"=0.0, "X Scale.Range:Maximum"=75.0, "Y Scale.Range:Minimum"=0.0, "Y Scale.Range:Maximum"=100.0) -> ()  [unwired: 2 in, 2 out]
          }
        }
        n2678 = case shown="True" "RST CP" {
          frame False {
          }
          frame True {
            n2679 = property on="Sample Temperature ( °C )" class="XYGraph (strict)"("Y Scale.Display Format:Precision"=u8 2 ("Y Scale.Format & Precision:Precision")) -> ()  [unwired: 2 in, 2 out]
            n2680 = property on="Sample Temperature ( °C )" class="XYGraph (strict)"("X Scale.Range:Minimum"=0.0, "X Scale.Range:Maximum"=75.0, "Y Scale.Range:Minimum"=58.0, "Y Scale.Range:Maximum"=62.0) -> ()  [unwired: 2 in, 2 out]
          }
        }
        n2681 = case shown="True" "RSTV1 3" {
          frame False {
          }
          frame True {
            n2682 = property on="Air Temperature  ( °C )" class="XYGraph (strict)"("Y Scale.Display Format:Precision"=u8 2 ("Y Scale.Format & Precision:Precision")) -> ()  [unwired: 2 in, 2 out]
            n2683 = property on="Air Temperature  ( °C )" class="XYGraph (strict)"("X Scale.Range:Minimum"=0.0 ("Y Scale.Range:Minimum"), "X Scale.Range:Maximum"=75.0 ("Y Scale.Range:Maximum"), "Y Scale.Range:Minimum"=20.0 ("X Scale.Range:Minimum"), "Y Scale.Range:Maximum"=26.0 ("X Scale.Range:Maximum")) -> ()  [unwired: 2 in, 2 out]
          }
        }
        n2684 = case shown="True" "RSTV1 4" {
          frame False {
          }
          frame True {
            n2685 = property on="Stroke ( mm )" class="XYGraph (strict)"("Y Scale.Display Format:Precision"=u8 2 ("Y Scale.Format & Precision:Precision")) -> ()  [unwired: 2 in, 2 out]
            n2686 = property on="Stroke ( mm )" class="XYGraph (strict)"("X Scale.Range:Minimum"=0.0 ("Y Scale.Range:Maximum"), "X Scale.Range:Maximum"=75.0 ("X Scale.Range:Minimum"), "Y Scale.Range:Minimum"=0.98, "Y Scale.Range:Maximum"=1.02) -> ()  [unwired: 2 in, 2 out]
          }
        }
        n2687 = case shown="True" "rstv2" {
          frame False {
          }
          frame True {
            n2688 = property on="Coefficient Of Friction" class="XYGraph (strict)"("Y Scale.Display Format:Precision"=u8 3 ("Y Scale.Format & Precision:Precision")) -> ()  [unwired: 2 in, 2 out]
            n2689 = property on="Coefficient Of Friction" class="XYGraph (strict)"("X Scale.Range:Minimum"=0.0 ("Y Scale.Range:Maximum"), "X Scale.Range:Maximum"=75.0, "Y Scale.Range:Minimum"=0.0, "Y Scale.Range:Maximum"=1.0 ("X Scale.Range:Minimum")) -> ()  [unwired: 2 in, 2 out]
          }
        }
        n2690 = case shown="True" "RST CP 3" {
          frame False {
          }
          frame True {
            n2691 = property on="Air Temp ( °C ) vs Humidity ( % RH )" class="XYGraph (strict)"("X Scale.Range:Minimum"=18.0, "X Scale.Range:Maximum"=28.0 ("X Scale.Range:Minimum"), "Y Scale.Range:Minimum"=30.0 ("X Scale.Range:Minimum"), "Y Scale.Range:Maximum"=70.0 ("X Scale.Range:Minimum")) -> ()  [unwired: 2 in, 2 out]
          }
        }
        n2692 = case shown="True" "OPEN 1" {
          frame False {
          }
          frame True {
            (unwired) 0  # existing file
            w3685 = "Choose a datalog file to open"  # prompt
            n2693 = local write "OPEN 1"(FALSE ("OPEN 1")) -> ()
            n2694 = String To Path(string="C:\\LAB-IQ\\Data\\") -> (path=w3670:path)
            n2695 = File Dialog(6:"*.dgf" ("pattern"), 7:w3685, 11:w3670) -> (0:w3668:errorcluster, 3:w3676:path)  [unwired: 4 in, 2 out]
            n2696 = Unbundle(w3668) -> ()  [unwired: 3 out]
            n2697 = Strip Path(path=w3676) -> (name=w3675:string)  [unwired: 1 out]
            n2698 = Path To String(path=w3676) -> (string=w3671:string)
            "string1" <- w3671
            n2699 = Match Pattern(string=w3675, regular expression=".dgf") -> (before substring=→"String Control":string)  [unwired: 1 in, 3 out]
            n2700 = Match Pattern(string=w3671, regular expression=".dgf" ("substring (\"\")")) -> (before substring=w3681:string)  [unwired: 1 in, 3 out]
            n2701 = Concatenate Strings(w3681, ".duf" ("Substring")) -> (w3677:string)
            n2702 = String To Path(string=w3677) -> (path=w3682:path)
            n2703 = call <vilib>:"Read Characters From File.vi"("file path (dialog if empty)"=w3682, "start of read offset (chars.:0)"=60 ("start of read offset (chars.: 0)")) -> ("character string"=→"String Control 2":string)  [unwired: 4 in, 3 out]
          }
        }
        n2704 = case shown="True" "OPEN 2" {
          frame False {
          }
          frame True {
            (unwired) 0  # existing file
            w3703 = "Choose a datalog file to open"  # prompt
            n2705 = local write "OPEN 2"(FALSE ("OPEN 1")) -> ()
            n2706 = String To Path(string="C:\\LAB-IQ\\Data\\") -> (path=w3688:path)
            n2707 = File Dialog(6:"*.dgf" ("pattern"), 7:w3703, 11:w3688) -> (0:w3686:errorcluster, 3:w3694:path)  [unwired: 4 in, 2 out]
            n2708 = Unbundle(w3686) -> ()  [unwired: 3 out]
            n2709 = Strip Path(path=w3694) -> (name=w3692:string)  [unwired: 1 out]
            n2710 = Path To String(path=w3694) -> (string=w3689:string)
            "string1 2" <- w3689
            n2711 = Match Pattern(string=w3692, regular expression=".dgf") -> (before substring=→"String Control 3":string)  [unwired: 1 in, 3 out]
            n2712 = Match Pattern(string=w3689, regular expression=".dgf" ("substring (\"\")")) -> (before substring=w3700:string)  [unwired: 1 in, 3 out]
            n2713 = Concatenate Strings(w3700, ".duf" ("Substring")) -> (w3697:string)
            n2714 = String To Path(string=w3697) -> (path=w3695:path)
            n2715 = call <vilib>:"Read Characters From File.vi"("file path (dialog if empty)"=w3695, "start of read offset (chars.:0)"=60 ("start of read offset (chars.: 0)")) -> ("character string"=→"String Control 4":string)  [unwired: 4 in, 3 out]
          }
        }
        n2716 = case shown="True" "OPEN 3" {
